vi "TMCM351-setSwitchdisable.vi"(4 "错误输入":errorcluster caption="错误输入（无错误）", 7 "com in":refnum<visa-resource-name>) -> (0 "错误输出":errorcluster, 3 "com out":refnum<visa-resource-name>)   [LabVIEW 2018]
uses:
  module_param.vi
panel:
  # "打开两个限位"
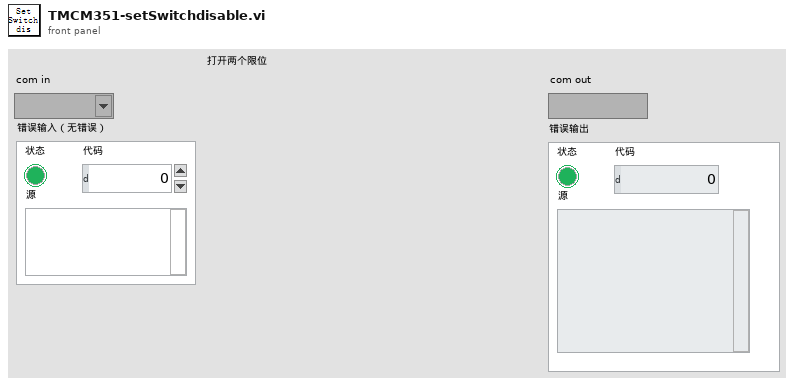
[diagram p1: front panel]
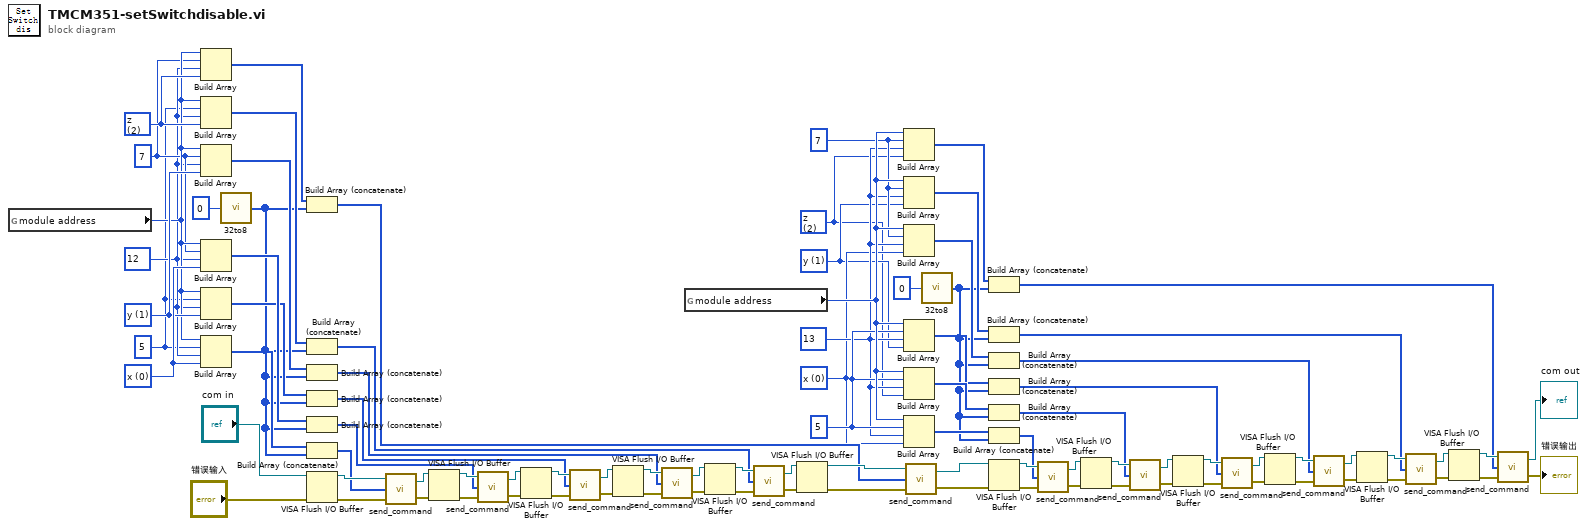
[diagram p0: block diagram]
diagram:
  w1 = u8 2 items=["x", "y", "z"] ("motor")
  w2 = u8 1 items=["x", "y", "z"] ("motor")
  w3 = u8 0 items=["x", "y", "z"] ("motor")
  w4 = u8 13
  w5 = u8 5 ("元素")
  w6 = u8 7 ("元素")
  w62 = u8 2 items=["x", "y", "z"] ("motor")
  w75 = u8 1 items=["x", "y", "z"] ("motor")
  w86 = u8 0 items=["x", "y", "z"] ("motor")
  w51 = u8 7 ("元素")
  w50 = u8 12
  w49 = u8 5
  n1 = global read "module_param.vi" "module address"() -> (w52:u8)
  n2 = Build Array(w52, w51, w50, w62) -> (w61:u8[])
  n3 = Build Array(w52, w49, w50, w62) -> (w64:u8[])
  n4 = Build Array(w52, w51, w50, w75) -> (w74:u8[])
  n5 = Build Array(w52, w51, w50, w86) -> (w85:u8[])
  n6 = Build Array(w52, w49, w50, w75) -> (w77:u8[])
  n7 = Build Array(w52, w49, w50, w86) -> (w88:u8[])
  n8 = call "32to8.vi"("32data_in"=0) -> ("8Array"=w53:u8[])
  n9 = Build Array (concatenate)(w61, w53) -> (w56:u8[])
  n10 = Build Array (concatenate)(w64, w53) -> (w63:u8[])
  n11 = Build Array (concatenate)(w74, w53) -> (w69:u8[])
  n12 = Build Array (concatenate)(w77, w53) -> (w76:u8[])
  n13 = Build Array (concatenate)(w85, w53) -> (w80:u8[])
  n14 = Build Array (concatenate)(w88, w53) -> (w87:u8[])
  n15 = VISA Flush I/O Buffer(VISA resource name="com in", error in (no error)="错误输入") -> (VISA resource name out=w90:refnum<visa-resource-name>, error out=w89:errorcluster)  [unwired: 1 in]
  n16 = call "send_command.vi"("错误输入"=w89, 3:w87, "com in"=w90) -> ("错误输出"=w83:errorcluster, "com out"=w84:refnum<visa-resource-name>)
  n17 = VISA Flush I/O Buffer(VISA resource name=w84, error in (no error)=w83) -> (VISA resource name out=w82:refnum<visa-resource-name>, error out=w81:errorcluster)  [unwired: 1 in]
  n18 = call "send_command.vi"("错误输入"=w81, 3:w80, "com in"=w82) -> ("错误输出"=w67:errorcluster, "com out"=w68:refnum<visa-resource-name>)
  n19 = VISA Flush I/O Buffer(VISA resource name=w68, error in (no error)=w67) -> (VISA resource name out=w79:refnum<visa-resource-name>, error out=w78:errorcluster)  [unwired: 1 in]
  n20 = call "send_command.vi"("错误输入"=w78, 3:w76, "com in"=w79) -> ("错误输出"=w72:errorcluster, "com out"=w73:refnum<visa-resource-name>)
  n21 = VISA Flush I/O Buffer(VISA resource name=w73, error in (no error)=w72) -> (VISA resource name out=w71:refnum<visa-resource-name>, error out=w70:errorcluster)  [unwired: 1 in]
  n22 = call "send_command.vi"("错误输入"=w70, 3:w69, "com in"=w71) -> ("错误输出"=w54:errorcluster, "com out"=w55:refnum<visa-resource-name>)
  n23 = global read "module_param.vi" "module address"() -> (w7:u8)
  n24 = VISA Flush I/O Buffer(VISA resource name=w55, error in (no error)=w54) -> (VISA resource name out=w66:refnum<visa-resource-name>, error out=w65:errorcluster)  [unwired: 1 in]
  n25 = call "send_command.vi"("错误输入"=w65, 3:w63, "com in"=w66) -> ("错误输出"=w59:errorcluster, "com out"=w60:refnum<visa-resource-name>)
  n26 = VISA Flush I/O Buffer(VISA resource name=w60, error in (no error)=w59) -> (VISA resource name out=w58:refnum<visa-resource-name>, error out=w57:errorcluster)  [unwired: 1 in]
  n27 = Build Array(w7, w6, w4, w1) -> (w21:u8[])
  n28 = Build Array(w7, w6, w4, w2) -> (w23:u8[])
  n29 = Build Array(w7, w6, w4, w3) -> (w33:u8[])
  n30 = Build Array(w7, w5, w4, w2) -> (w35:u8[])
  n31 = Build Array(w7, w5, w4, w1) -> (w43:u8[])
  n32 = Build Array(w7, w5, w4, w3) -> (w45:u8[])
  n33 = call "send_command.vi"("错误输入"=w57, 3:w56, "com in"=w58) -> ("错误输出"=w10:errorcluster, "com out"=w11:refnum<visa-resource-name>)
  n34 = call "32to8.vi"("32data_in"=0) -> ("8Array"=w13:u8[])
  n35 = Build Array (concatenate)(w21, w13) -> (w16:u8[])
  n36 = Build Array (concatenate)(w23, w13) -> (w22:u8[])
  n37 = Build Array (concatenate)(w33, w13) -> (w28:u8[])
  n38 = Build Array (concatenate)(w35, w13) -> (w34:u8[])
  n39 = Build Array (concatenate)(w43, w13) -> (w38:u8[])
  n40 = Build Array (concatenate)(w45, w13) -> (w44:u8[])
  n41 = VISA Flush I/O Buffer(VISA resource name=w11, error in (no error)=w10) -> (VISA resource name out=w47:refnum<visa-resource-name>, error out=w46:errorcluster)  [unwired: 1 in]
  n42 = call "send_command.vi"("错误输入"=w46, 3:w44, "com in"=w47) -> ("错误输出"=w41:errorcluster, "com out"=w42:refnum<visa-resource-name>)
  n43 = VISA Flush I/O Buffer(VISA resource name=w42, error in (no error)=w41) -> (VISA resource name out=w40:refnum<visa-resource-name>, error out=w39:errorcluster)  [unwired: 1 in]
  n44 = call "send_command.vi"("错误输入"=w39, 3:w38, "com in"=w40) -> ("错误输出"=w26:errorcluster, "com out"=w27:refnum<visa-resource-name>)
  n45 = VISA Flush I/O Buffer(VISA resource name=w27, error in (no error)=w26) -> (VISA resource name out=w37:refnum<visa-resource-name>, error out=w36:errorcluster)  [unwired: 1 in]
  n46 = call "send_command.vi"("错误输入"=w36, 3:w34, "com in"=w37) -> ("错误输出"=w31:errorcluster, "com out"=w32:refnum<visa-resource-name>)
  n47 = VISA Flush I/O Buffer(VISA resource name=w32, error in (no error)=w31) -> (VISA resource name out=w30:refnum<visa-resource-name>, error out=w29:errorcluster)  [unwired: 1 in]
  n48 = call "send_command.vi"("错误输入"=w29, 3:w28, "com in"=w30) -> ("错误输出"=w14:errorcluster, "com out"=w15:refnum<visa-resource-name>)
  n49 = VISA Flush I/O Buffer(VISA resource name=w15, error in (no error)=w14) -> (VISA resource name out=w25:refnum<visa-resource-name>, error out=w24:errorcluster)  [unwired: 1 in]
  n50 = call "send_command.vi"("错误输入"=w24, 3:w22, "com in"=w25) -> ("错误输出"=w19:errorcluster, "com out"=w20:refnum<visa-resource-name>)
  n51 = VISA Flush I/O Buffer(VISA resource name=w20, error in (no error)=w19) -> (VISA resource name out=w18:refnum<visa-resource-name>, error out=w17:errorcluster)  [unwired: 1 in]
  n52 = call "send_command.vi"("错误输入"=w17, 3:w16, "com in"=w18) -> ("错误输出"=→"错误输出":errorcluster, "com out"=→"com out":refnum<visa-resource-name>)
